vi "4_1.vi"() -> ()   [LabVIEW 2020]
panel:
  out "Array 3":i32[][](array[numeric])
  out "Array 2":dbl[][](array[numeric])
  out "Array":i32[][](array[numeric])
  in  "Num of row":i32
  in  "Num of column":i32
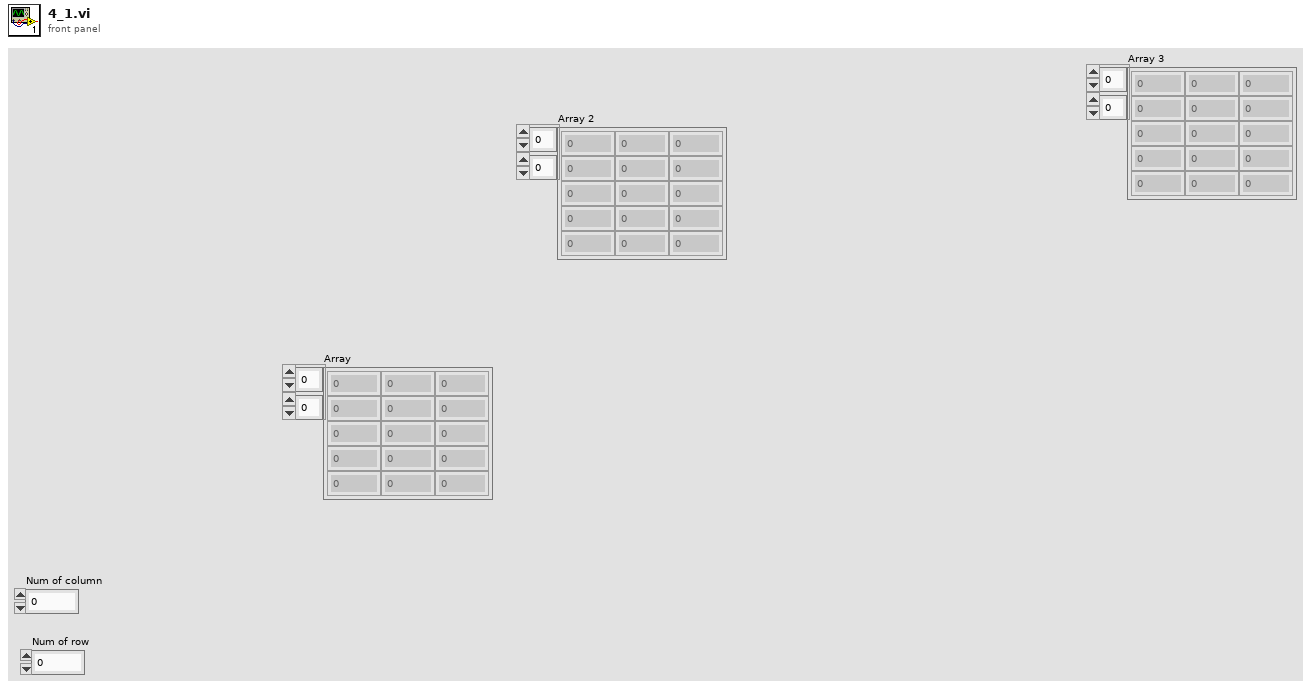
[diagram p1: front panel]
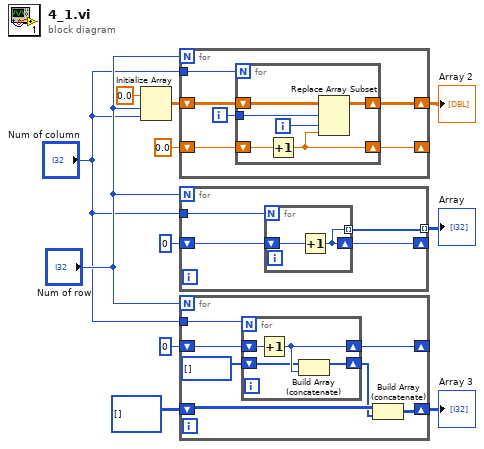
[diagram p0: block diagram]
diagram:
  n1 = Initialize Array(0.0 ("element"), "Num of row", "Num of column") -> (w9:dbl[][])
  n2 = for {
    N: "Num of row" -> [_]
    shift-right: [w16] -> w6
    shift-left: w9 -> [w17]
    shift-right: [w13] -> _
    shift-left: 0.0 -> [w14]
    tunnel: "Num of column" -> [w12]
    i -> [w15]
    n3 = for {
      N: w12 -> [_]
      shift-right: [w22] -> w16
      shift-left: w17 -> [w23]
      tunnel: w15 -> [w21]
      shift-right: [w18] -> w13
      shift-left: w14 -> [w19]
      i -> [w20]
      n4 = Increment(x=w19) -> (x+1=w18:dbl)
      n5 = Replace Array Subset(array=w23, new element=w18, index (row)=w21, index (col)=w20) -> (w22:dbl[][])
    }
  }
  "Array 2" <- w6
  n6 = for {
    N: "Num of row" -> [_]
    shift-right: [w27] -> _
    shift-left: 0 -> [w26]
    tunnel: [w25] -> w10 mode=indexing
    tunnel: "Num of column" -> [w24]
    n7 = for {
      N: w24 -> [_]
      shift-right: [w28] -> w27
      shift-left: w26 -> [w29]
      tunnel: [w28] -> w25 mode=indexing
      n8 = Increment(x=w29) -> (x+1=w28:i32)
    }
  }
  "Array" <- w10
  n9 = for {
    N: "Num of row" -> [_]
    shift-right: [w36] -> _
    shift-left: 0 -> [w35]
    tunnel: "Num of column" -> [w34]
    shift-right: [w33] -> w1
    shift-left: i32[][] [] -> [w31]
    n10 = for {
      N: w34 -> [_]
      shift-right: [w39] -> w36
      shift-left: w35 -> [w40]
      shift-right: [w38] -> w30
      shift-left: i32[] [] -> [w37]
      n11 = Increment(x=w40) -> (x+1=w39:i32)
      n12 = Build Array (concatenate)(w37, w39) -> (w38:i32[])
    }
    n13 = Build Array (concatenate)(w31, w30) -> (w33:i32[][])
  }
  "Array 3" <- w1
